vi "Number of Periods.vi"(8 "error in (no error)":errorcluster, 10 "# of periods (def: 1)":i32=1 min=0 max=2000 step=1, 11 "VISA resource name":refnum<visa-resource-name>) -> (0 "error out":errorcluster, 3 "VISA resource name out":refnum<visa-resource-name>)   [LabVIEW 2012, in "SR400.lvlib"]
doc: "NP { m }\nIf m is absent, the NP command returns the\nprogrammed number of periods in a scan (N\nPERIODS). If m is included, the number of\nperiods is set to the value m. The parameter m\nmust be an integer from 1 to 2000. Changing the\nnumber of periods during a scan is allowed. If the\nnew value exceeds the current scan position, then\nthe scan will continue to the new number of\nperiods. If the new value is lower than the current\nscan position, then the scan ends at the next end of\ncount period."
uses:
  SR400.lvlib
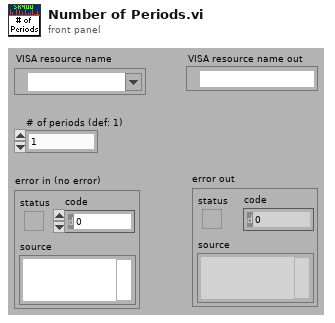
[diagram p1: front panel]
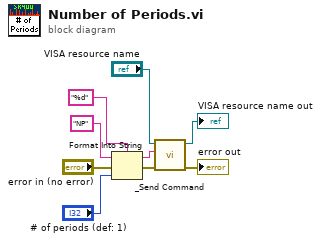
[diagram p0: block diagram]
diagram:
  n1 = Format Into String(format string="%d", initial string="NP" ("command"), error in="error in (no error)", "# of periods (def: 1)") -> (resulting string=w4:string, error out=w3:errorcluster)
  n2 = call "_Send Command.vi"("error in (no error)"=w3, "Command"=w4, "VISA resource name"="VISA resource name") -> ("error out"=→"error out":errorcluster, "VISA resource name out"=→"VISA resource name out":refnum<visa-resource-name>)  [unwired: 1 in, 6 out]
